vi "Log Action.vi"(4 "Log Map in":refnum<class "LogMap.lvclass">, 8 "error in (no error)":errorcluster, 9 "object in":refnum<class>, 10 "ActionType":string, 11 "SqlMapper in":refnum<class "SqlMapper.lvclass">) -> (0 "error out":errorcluster, 3 "SqlMapper out":refnum<class "SqlMapper.lvclass">)   [LabVIEW 2020, in "ORM.lvlib" / "LogMap.lvclass"]
uses:
  LogMap.lvclass
  C:/Viviota/Projects/R&D/__OpenSource/VIV_ORM/ORM/TypeMap/TypeMap.lvclass
  SqlMapper/SqlMapper.lvclass
  LogMap.lvclass/LogMap.ctl
  TypeMap/TypeMap.lvclass
  TypeMap/TypeMap.lvclass/TypeMap.ctl
  TypeMap/Read Autokey.vi
  Read IncludeObjRepresentation.vi
  Read XtraJsonEncodeObj.vi
  TypeMap/Write ExplicitFieldOrder.vi
  TypeMap/Read Table Name.vi
  TypeMap/Write Table Name.vi
  <vilib>/JDP Science/JSONtext/JSONtext.lvlib
  <vilib>/Viviota/shared/ORM_lib.lvlibp/ObjectRow/ObjectLUT.lvclass
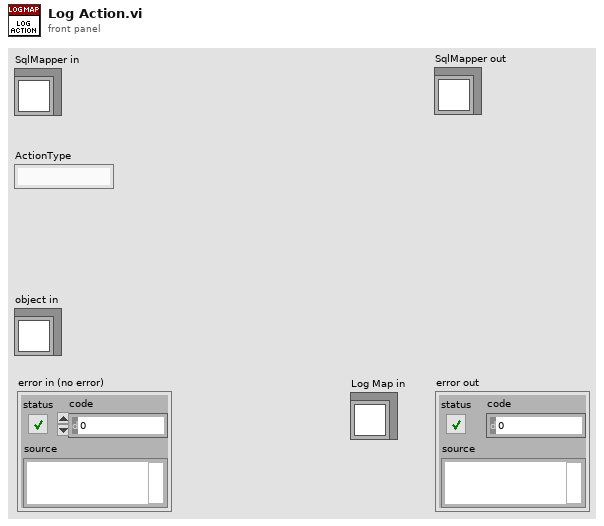
[diagram p1: front panel]
types:
  T1 = typedef "ORM.lvlib/LogMap.lvclass/logmapcluster.ctl" = cluster{"ActionTime":timestamp, "ActionType":string, "ObjectTable":string, "ObjectId":i64, "ObjectRepr":string, "Username":string, "Domain":string, "IP":string, "MachineGuid":string}
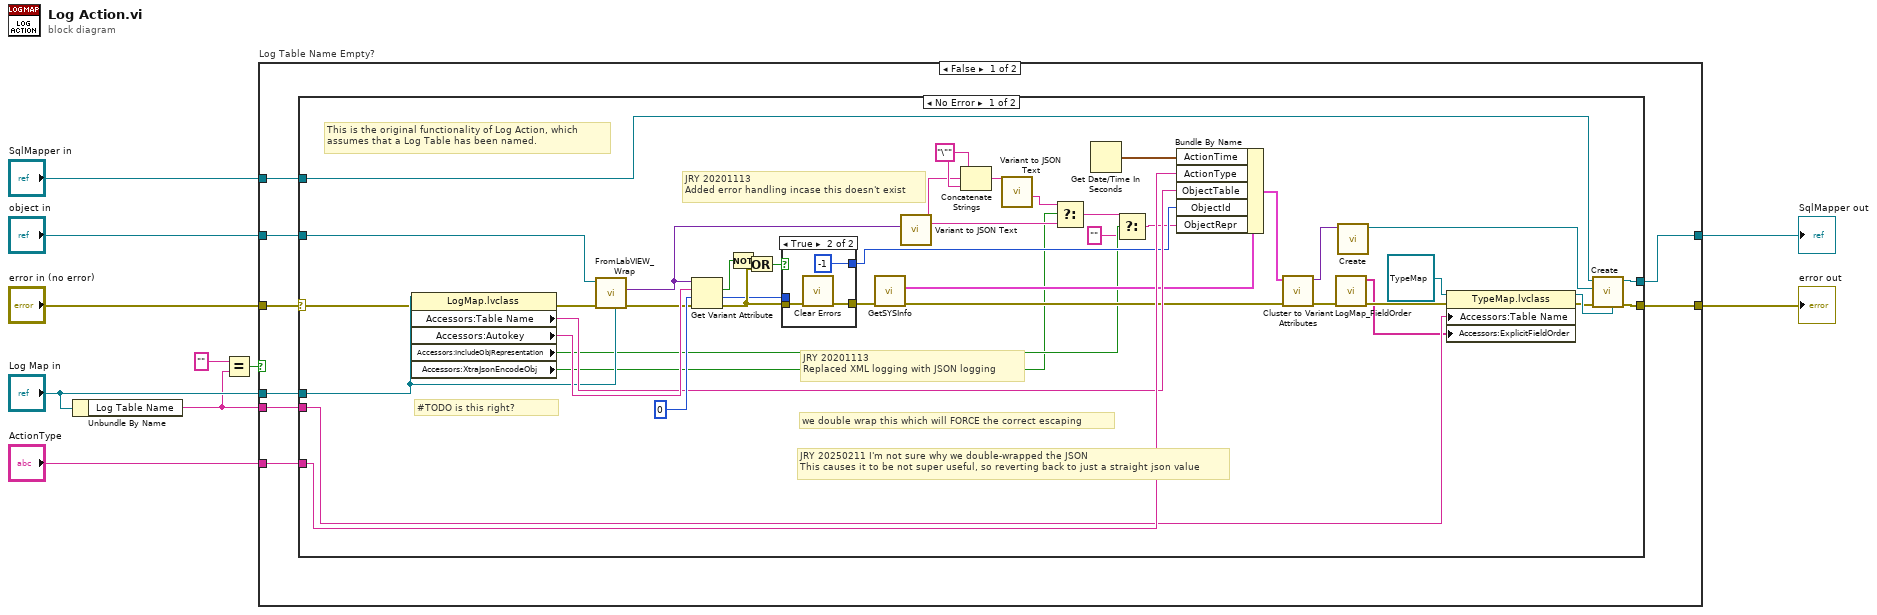
[diagram p0: block diagram]
diagram:
  n1 = Unbundle By Name("Log Map in") -> ("Log Table Name"=w1:string)
  n2 = Equal?(x="", y=w1) -> (x = y?=w2:bool)
  n3 = case "Log Table Name Empty?" shown="False" w2 {
    tunnel: "ActionType" -> [w18 _]
    tunnel: "object in" -> [w17 _]
    tunnel: [w16 w69] -> w8
    tunnel: "SqlMapper in" -> [w15 w69]
    tunnel: [w14 w68] -> w6
    tunnel: "error in (no error)" -> [w13 w68]
    tunnel: "Log Map in" -> [w12 _]
    tunnel: w1 -> [w11 _]
    frame False {
      n4 = case shown="No Error" w13 {
        selector: w13 -> [w36 w67]
        tunnel: w12 -> [w51 _]
        tunnel: w17 -> [w52 _]
        tunnel: w15 -> [w29 w66]
        tunnel: [w60 w67] -> w14
        tunnel: [w59 w66] -> w16
        tunnel: w18 -> [w56 _]
        tunnel: w11 -> [w45 _]
        frame No Error {
          w34 = "\"" ("string")
          # "JRY 20250211 I'm not sure why we double-wrapped the JSON\nThis causes it to be not super useful, so reverting back to just a straight json value"
          # "we double wrap this which will FORCE the correct escaping"
          # "JRY 20201113\nAdded error handling incase this doesn't exist"
          # "JRY 20201113 \nReplaced XML logging with JSON logging"
          # "This is the original functionality of Log Action, which \nassumes that a Log Table has been named."
          # "#TODO is this right?"
          n5 = property class="LogMap.lvclass"(reference=w51, error in=w36) -> (error out=w49:errorcluster, "Accessors:Table Name"=w53:string, "Accessors:Autokey"=w55:string, "Accessors:IncludeObjRepresentation"=w25:bool, "Accessors:XtraJsonEncodeObj"=w19:bool)  [unwired: 1 out]
          n6 = call "FromLabVIEW_Wrap.vi"("TypeMap in"=w51, "error in (no error)"=w49, "object in"=w52) -> ("error out"=w50:errorcluster, "DbRow"=w44:variant)  [unwired: 7 in]
          n7 = Get Variant Attribute(Variant=w44, name=w55, default value (empty Variant)=i64 0 ("ObjectId"), error in=w50) -> (found=w43:bool, value=w38:i64, error out=w40:errorcluster)  [unwired: 1 out]
          n8 = Not(x=w43) -> (.not. x?=w42:bool)
          n9 = Or(x=w42, y=w40) -> (x .or. y?=w41:bool)
          n10 = case shown="True" w41 {
            tunnel: w40 -> [w61 w64]
            tunnel: [w62 -1] -> w39
            tunnel: w38 -> [w62 _]
            tunnel: [w61 w63] -> w37
            frame False {
            }
            frame True {
              n11 = call <vilib>:"Clear Errors.vi"("error in (no error)"=w64) -> ("error out"=w63:errorcluster)  [unwired: 5 in, 1 out]
            }
          }
          n12 = call "GetSYSInfo.vi"("error in (no error)"=w37) -> ("error out"=w48:errorcluster, "Info"=w33:T1)  [unwired: 9 in]
          n13 = call <vilib>:"Variant to JSON Text.vi"("Variant"=w44) -> ("<JSON>"=w20:string)  [unwired: 8 in, 2 out]
          n14 = Concatenate Strings(w34, w20, w34) -> (w23:string)
          n15 = call <vilib>:"Variant to JSON Text.vi"("Variant"=w23) -> ("Name of data in Variant"=w22:string)  [unwired: 8 in, 2 out]
          n16 = Select(t=w22, s=w19, f=w20) -> (s? t:f=w21:string)
          n17 = Get Date/Time In Seconds() -> (seconds since 1Jan1904=w35:timestamp)
          n18 = Select(t=w21, s=w25, f="") -> (s? t:f=w26:string)
          n19 = Bundle By Name(cluster=w33, "ActionTime"=w35, "ActionType"=w56, "ObjectTable"=w53, "ObjectId"=w39, "ObjectRepr"=w26) -> (w46:T1)
          n20 = call "Cluster to Variant Attributes.vi"("error in (no error)"=w48, "Cluster"=w46) -> ("error out"=w32:errorcluster, "Variant"=w28:variant)  [unwired: 8 in]
          n21 = call "LogMap_FieldOrder.vi"("Error In"=w32) -> ("Error Out"=w31:errorcluster, "FieldOrder out"=w30:string[])  [unwired: 9 in]
          n22 = call <vilib>:"Create.vi"("LUT"=w28) -> ("ORM_lib.lvlib:ObjectLUT.lvclass"=w27:refnum<class "ObjectLUT.lvclass">)  [unwired: 9 in, 1 out]
          n23 = property class="TypeMap.lvclass"(reference=refnum<class "TypeMap.lvclass"> refnum ("TypeMap in"), error in=w31, "Accessors:Table Name"=w45, "Accessors:ExplicitFieldOrder"=w30) -> (reference out=w57:refnum<class "TypeMap.lvclass">, error out=w47:errorcluster)
          n24 = call-dynamic <vilib>:"Create.vi"("TypeMap in"=w57, "error in (no error)"=w47, "object in"=w27, "SqlMapper in"=w29) -> ("error out"=w60:errorcluster, "SqlMapper out"=w59:refnum<class "SqlMapper.lvclass">)  [unwired: 4 in, 2 out]
        }
        frame Error {
        }
      }
    }
    frame True {
      # "When the Log Table name is an empty string, \nthen no logging action will occur."
    }
  }
  "SqlMapper out" <- w8
  "error out" <- w6
